vi "Read Source.vi"(8 "error in (no error)":errorcluster, 11 "Target in":refnum<class "Target.lvclass">) -> (0 "error out":errorcluster, 2 "Source":T3, 3 "Target out":refnum<class "Target.lvclass">)   [LabVIEW 2015, in "Target.lvclass"]
uses:
  Target.lvclass
  XML Controls/Path Cluster.ctl
  XML Controls/Target.ctl
  Target.lvclass/Target.ctl
  Configuration Tool.lvlib
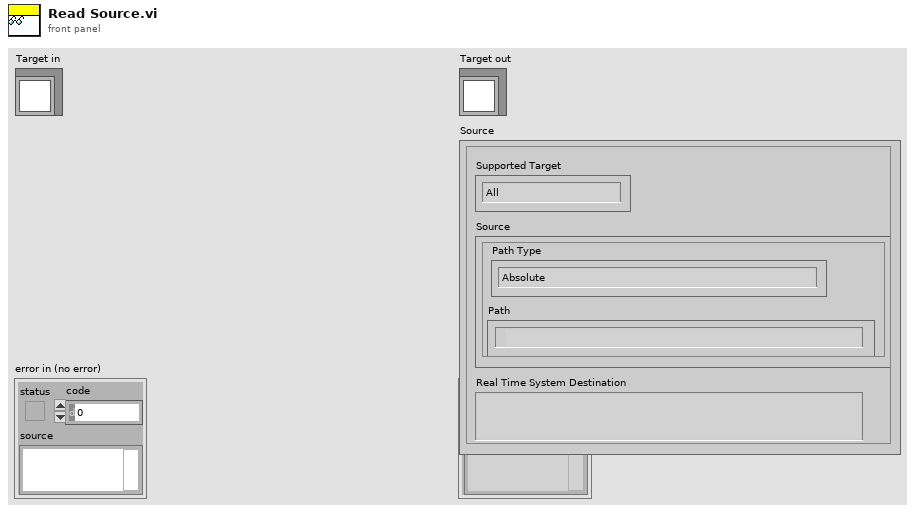
[diagram p1: front panel]
types:
  T1 = typedef "Configuration Tool.lvlib/Path Cluster.ctl" = cluster{"Path":path, "Path Type":enum16{"Absolute", "To Base", "To Common Doc Dir", "To Application Data Dir"}}
  T2 = typedef "Configuration Tool.lvlib/Target.ctl" = enum16{"All", "Pharlap", "VxWorks", "Windows", "Linux_32_ARM", "Linux_x64", "PharlapWindows", "PharlapVxWorks", "VxWorksWindows"}
  T3 = cluster{"Source":T1, "Real Time System Destination":string, "Supported Target":T2}
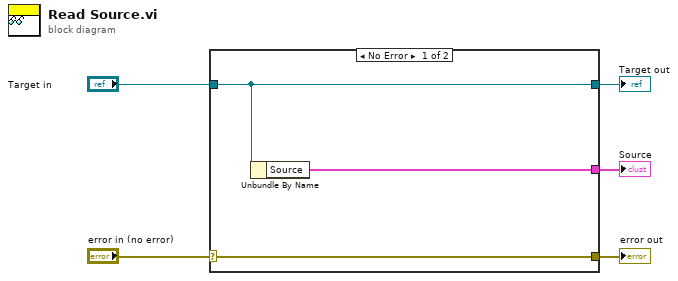
[diagram p0: block diagram]
diagram:
  n1 = case shown="No Error" "error in (no error)" {
    selector: "error in (no error)" -> [w8 w9]
    tunnel: [w8 w9] -> w4
    tunnel: [w7 w10] -> w2
    tunnel: "Target in" -> [w7 w10]
    tunnel: [w6 _] -> w1
    frame No Error {
      n2 = Unbundle By Name(w7) -> ("Source"=w6:T3)
    }
    frame Error {
    }
  }
  "error out" <- w4
  "Target out" <- w2
  "Source" <- w1
